vi "Login - Developer Mode.vi"(8 "Error In":errorcluster) -> (0 "Error Out":errorcluster, 3 "Login?":bool)   [LabVIEW 2020]
uses:
  <vilib>/Utility/miscctls.llb/LVPositionTypeDef.ctl
  Control/State - FGV.ctl
  <vilib>/picture/picture.llb/imagedata.ctl
panel:
  out "BG Image":picture
  in  "Cancel":bool
  in  "Login":bool
  in  "Password:":string
  in  "Username:":string
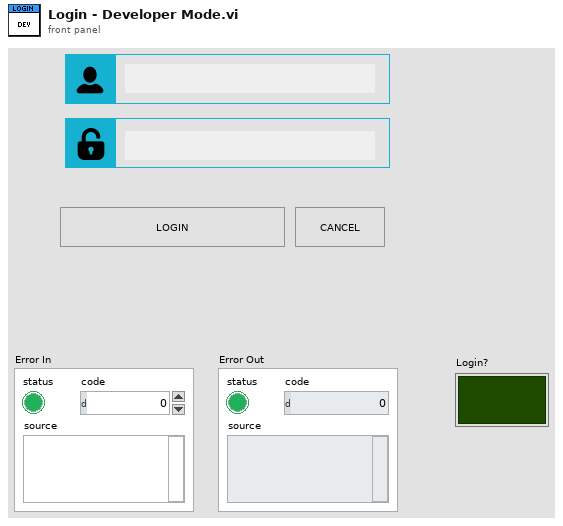
[diagram p1: front panel]
types:
  T1 = typedef "State - FGV.ctl" = enum16{"Write", "Read"}
  T2 = typedef "LVPositionTypeDef.ctl" = cluster{"Left":i32, "Top":i32}
  T3 = typedef "imagedata.ctl" = cluster{"image type":i32, "image depth":i32, "image":u8[], "mask":u8[], "colors":u32[], "Rectangle":cluster{"left":i16, "top":i16, "right":i16, "bottom":i16}}
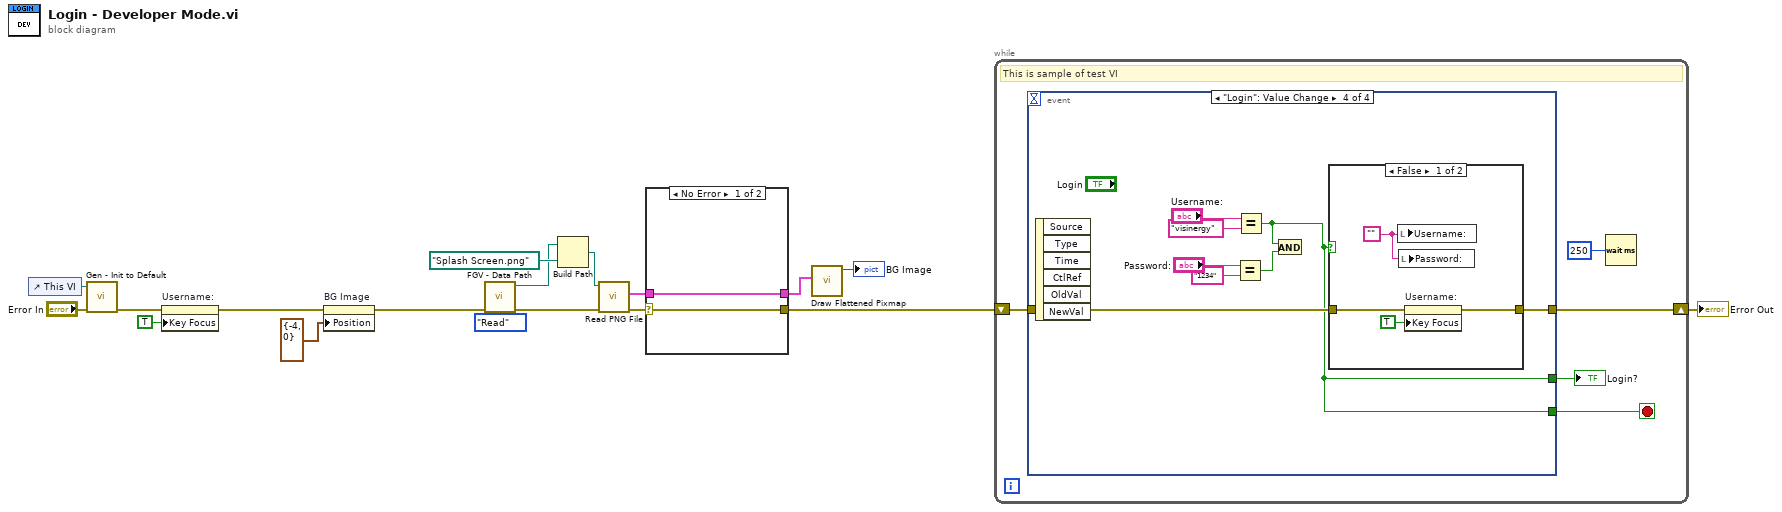
[diagram p0: block diagram]
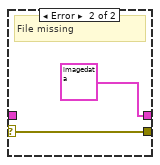
[diagram p2: hidden frame]
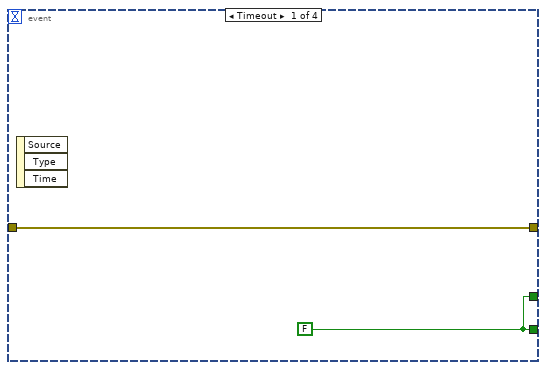
[diagram p3: hidden frame]
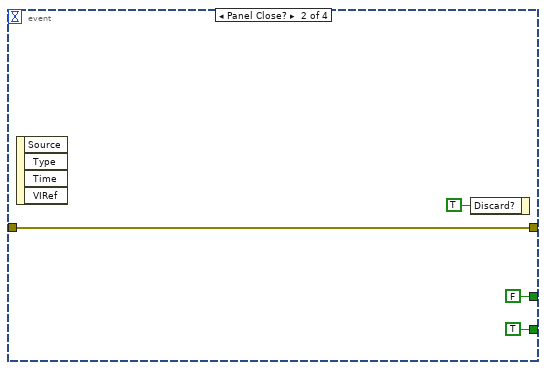
[diagram p4: hidden frame]
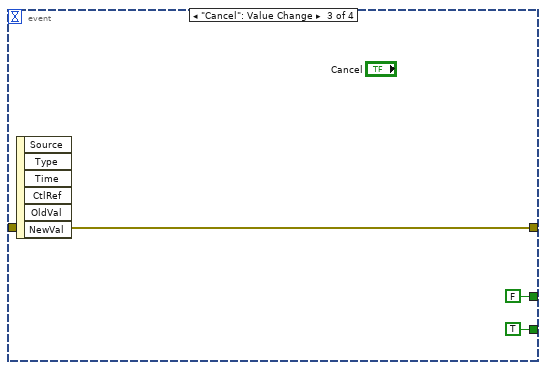
[diagram p5: hidden frame]
diagram:
  n1 = control-ref of="This VI"() -> (w15:refnum<vi>)
  n2 = call "Gen - Init to Default.vi"("Error in"="Error In", "This VI"=w15) -> ("Error out"=w17:errorcluster)  [unwired: 8 in, 1 out]
  n3 = property on="Username:" class="Str"(error in=w17, "Key Focus"=TRUE) -> (error out=w12:errorcluster)  [unwired: 1 in, 1 out]
  n4 = property on="BG Image" class="Pict"(error in=w12, "Position"=T2 {"Left"=-4, "Top"=0}) -> (error out=w4:errorcluster)  [unwired: 1 in, 1 out]
  n5 = call "FGV - Data Path.vi"("FGV State"=State_-_FGV."Read", "Error In"=w4) -> ("Error Out"=w2:errorcluster, "Path Out"=w5:path)  [unwired: 8 in]
  n6 = Build Path(base path=w5, name or relative path=path "Splash Screen.png") -> (appended path=w11:path)
  n7 = call <vilib>:"Read PNG File.vi"("error in (no error)"=w2, "path to PNG file"=w11) -> ("error out"=w8:errorcluster, "image data"=w7:T3)  [unwired: 7 in, 1 out]
  n8 = case shown="No Error" w8 {
    selector: w8 -> [w20 w21]
    tunnel: [w20 w21] -> w1
    tunnel: [w19 T3 {"image type"=0, "image depth"=32, "image"=array[1013796 elements], "mask"=array[32184 elements], "colors"=[], "Rectangle"={"left"=0, "top"=0, "right"=567, "bottom"=447}} ("image data")] -> w6
    tunnel: w7 -> [w19 _]
    frame No Error {
    }
    frame Error {
      # "File missing"
    }
  }
  n9 = call <vilib>:"Draw Flattened Pixmap.vi"("image data"=w6) -> ("new picture"=→"BG Image":picture)  [unwired: 8 in]
  n10 = while {
    shift-right: [w27] -> w18
    shift-left: w1 -> [w26]
    stop <- w24 stop-if-true
    # "This is sample of test VI"
    n11 = event shown="[3] \"Login\": Value Change" {
      selector: _ -> [_ _ _ _]
      dyn-events: _ -> [_ _ _ _]
      timeout: _ -> [_ _ _ _]
      tunnel: [w29 w33 w36 w43] -> w27
      tunnel: w26 -> [w29 w33 w36 w44]
      tunnel: [w28 TRUE TRUE w37] -> w24
      tunnel: [w28 FALSE FALSE w37] -> w23
      event Timeout {
        w28 = FALSE
        n12 = event-data() -> ()  [unwired: 1 in, 3 out]
      }
      event Panel Close? {
        n13 = event-data() -> ()  [unwired: 1 in, 4 out]
        n14 = event-data("Discard?"=TRUE) -> ()  [unwired: 1 in, 1 out]
      }
      event "Cancel": Value Change {
        n15 = event-data() -> ()  [unwired: 1 in, 6 out]
      }
      event "Login": Value Change {
        n16 = event-data() -> ()  [unwired: 1 in, 6 out]
        n17 = Equal?(x="Password:", y="1234") -> (x = y?=w38:bool)
        n18 = Equal?(x="Username:", y="visinergy") -> (x = y?=w37:bool)
        n19 = And(x=w37, y=w38) -> ()  [unwired: 1 out]
        n20 = case shown="False" w37 {
          tunnel: w44 -> [w48 w49]
          tunnel: [w47 w49] -> w43
          frame False {
            w46 = ""
            n21 = local write "Username:"(w46) -> ()
            n22 = local write "Password:"(w46) -> ()
            n23 = property on="Username:" class="Str"(error in=w48, "Key Focus"=TRUE) -> (error out=w47:errorcluster)  [unwired: 1 in, 1 out]
          }
          frame True {
          }
        }
      }
    }
    "Login?" <- w23
    n24 = Wait (ms)(milliseconds to wait=u32 250) -> ()  [unwired: 1 out]
  }
  "Error Out" <- w18
